vi "Replace Control in VI (Scalar).vi"(8 "error in":errorcluster, 10 "Control Replacement Params":T1, 11 "Original VI":path=path "C:/Users/OneEd/OneDrive/Desktop/MicroPort Job/CTDB/src/db_script/DB Select Template.vi") -> (0 "error out":errorcluster, 3 "Save as out":path=path "C:/Users/OneEd/OneDrive/Desktop/MicroPort Job/CTDB/src/db_script/DB Select Template.vi")   [LabVIEW 2022 SP3, in "EDT VI Script.lvlib"]
uses:
  EDT VI Script.lvlib
  Control Replacement Param.ctl
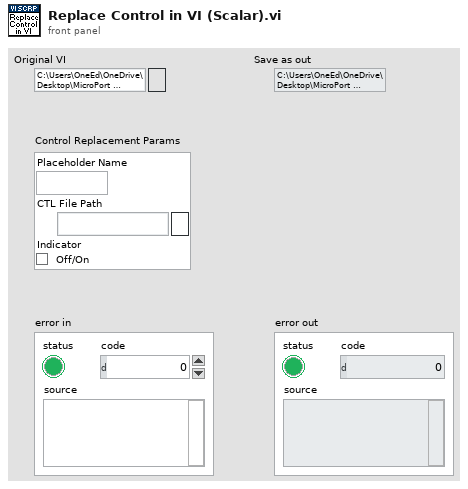
[diagram p1: front panel]
types:
  T1 = typedef "EDT VI Script.lvlib/Control Replacement Param.ctl" = cluster{"Placeholder Name":string, "CTL File Path":path, "Indicator":bool}
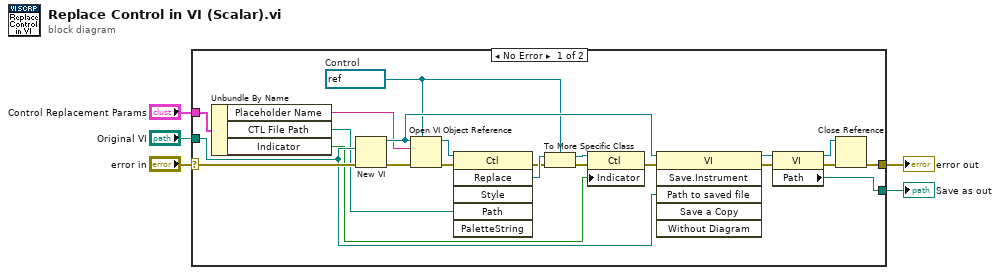
[diagram p0: block diagram]
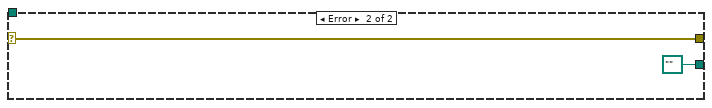
[diagram p2: hidden frame]
diagram:
  n1 = case shown="No Error" "error in" {
    selector: "error in" -> [w27 w29]
    tunnel: [w24 w29] -> w4
    tunnel: "Original VI" -> [w16 _]
    tunnel: "Control Replacement Params" -> [w25 _]
    tunnel: [w20 path "" ("Path")] -> w1
    frame No Error {
      w9 = refnum<vi> refnum  # Control
      n2 = Unbundle By Name(w25) -> ("Placeholder Name"=w15:string, "CTL File Path"=w13:path, "Indicator"=w12:bool)
      n3 = New VI(8:w27, 10:w16) -> (0:w26:errorcluster, 3:w23:refnum<vi>)  [unwired: 5 in]
      n4 = Open VI Object Reference(7:w9, 8:w26, 10:w15, 11:w23) -> (0:w11:errorcluster, 3:w14:refnum<vi>)
      n5 = invoke on="Invoke Node" class="Ctl" method="Replace"(reference=w14, error in=w11, "Path"=w13) -> (error out=w7:errorcluster, "Replace"=w10:refnum<vi>)  [unwired: 3 in, 4 out]
      n6 = To More Specific Class(target class=w9, reference=w10, error in=w7) -> (specific class reference=w8:refnum<vi>, error out=w6:errorcluster)
      n7 = property class="Ctl"(reference=w8, error in=w6, "Indicator"=w12) -> (error out=w19:errorcluster)  [unwired: 1 out]
      n8 = invoke class="VI" method="Save.Instrument"(reference=w23, error in=w19, "Path to saved file"=w16) -> (reference out=w18:refnum<vi>, error out=w17:errorcluster)  [unwired: 3 in, 4 out]
      n9 = property class="VI"(reference=w18, error in=w17) -> (reference out=w22:refnum<vi>, error out=w21:errorcluster, "Path"=w20:path)
      n10 = Close Reference(reference=w22, error in (no error)=w21) -> (error out=w24:errorcluster)
    }
    frame Error {
    }
  }
  "error out" <- w4
  "Save as out" <- w1
